vi "LucaStartAcquisition.vi"(5 "Camera Index":i32=1, 6 "Continuous":bool=TRUE, 7 "input cluster":T1={"left"=1, "right"=-1, "top"=1, "bottom"=-1}, 8 "error in (no error) 2":errorcluster, 9 "Bin Size":i32=1, 10 "EMCCD Gain":i32=200, 11 "Exposure Time":sgl=0.3 format="%.2f") -> (0 "error out":errorcluster={"status"=FALSE, "code"=0, "source"="LucaDetectIon.vi->LucaStartAcquisition.vi->SetShutter.vi"}, 3 "Image":u16[][](array[numeric]))   [LabVIEW 2009]
uses:
  <userlib>/atmcd32d.llb/AcquisitionMode_mode typedef.ctl
  <userlib>/atmcd32d.llb/ReadMode_mode typedef.ctl
  <userlib>/atmcd32d.llb/TriggerMode_mode typedef.ctl
  <userlib>/atmcd32d.llb/Shutter_mode typedef.ctl
  <userlib>/atmcd32d.llb/Shutter_type typedef.ctl
panel:
  out "Calculated Exposure Time":sgl=0.3 format="%.2f"
  out "Kinetic Cycle Time":sgl=0.3009 format="%.2f"
  out "Accumulate Time":sgl=0.3009 format="%.2f"
  out "Set Trigger Mode\nError Code":u32=20002
  out "Camera Serial":i32=1151
  out "Initialize Error Code":u32=20002
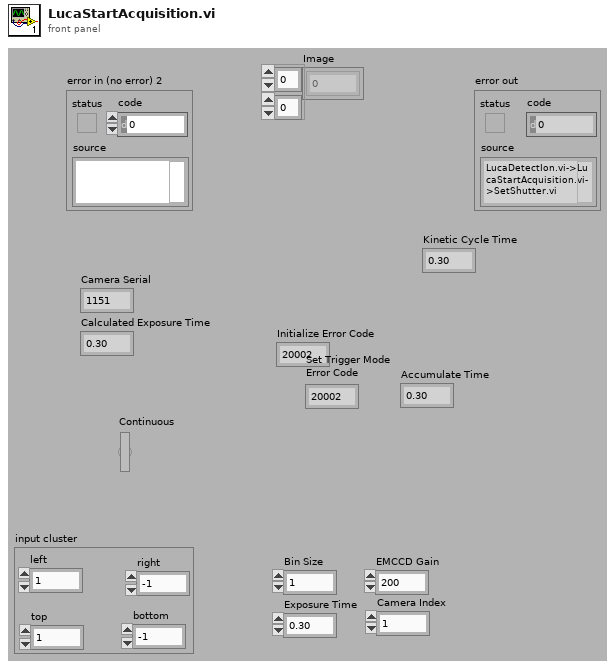
[diagram p1: front panel]
types:
  T1 = cluster{"left":i32, "right":i32, "top":i32, "bottom":i32}
  T2 = typedef "AcquisitionMode_mode typedef.ctl" = enum16{"Reserved (0)", "Single Scan", "Accumulate", "Kinetics", "Fast Kinetics", "Run Till Abort", "Reserved (6)", "Reserved (7)", "Reserved (8)", "Time Delayed Integration"}
  T3 = typedef "ReadMode_mode typedef.ctl" = enum16{"Full Vertical Binning", "Multi-Track", "Random-Track", "Single-Track", "Image"}
  T4 = typedef "TriggerMode_mode typedef.ctl" = enum16{"Internal", "External", "N/A (2)", "N/A (3)", "N/A (4)", "N/A (5)", "External Start"}
  T5 = typedef "Shutter_mode typedef.ctl" = enum16{"Auto", "Open", "Close"}
  T6 = typedef "Shutter_type typedef.ctl" = enum16{"TTL Low", "TTL High"}
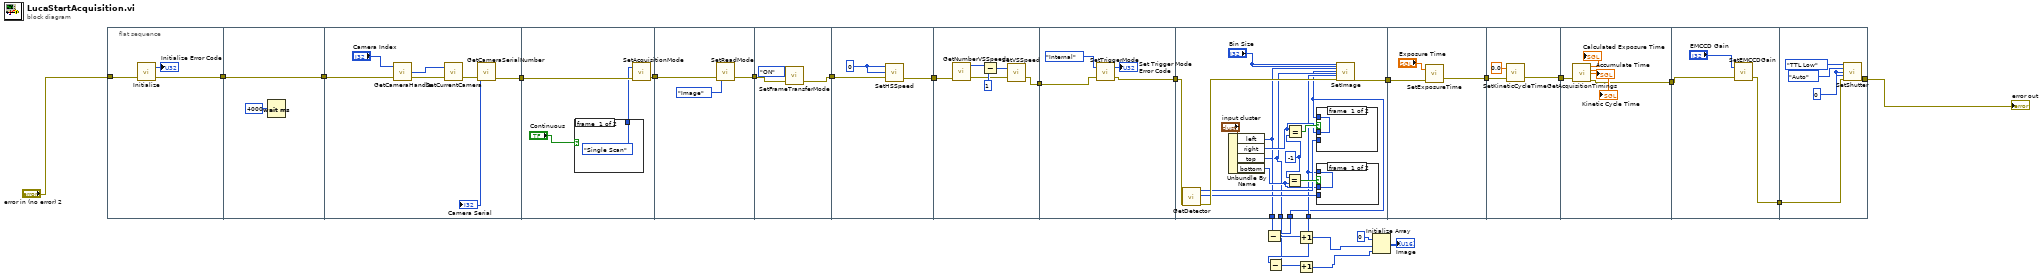
[diagram p0: block diagram]
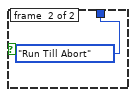
[diagram p2: hidden frame]
diagram:
  n1 = flat-sequence {
    tunnel: [w28] -> w26
    tunnel: "error in (no error) 2" -> [w27]
    tunnel: [w30] -> w25
    tunnel: w26 -> [w30]
    tunnel: [w33] -> w24
    tunnel: w25 -> [w32]
    tunnel: w24 -> [w42]
    tunnel: [w41] -> w23
    tunnel: w23 -> [w46]
    tunnel: [w45] -> w6
    tunnel: w6 -> [w50]
    tunnel: [w49] -> w5
    tunnel: w5 -> [w52]
    tunnel: [w51] -> w22
    tunnel: w22 -> [w56]
    tunnel: [w54] -> w21
    tunnel: w21 -> [w60]
    tunnel: [w61] -> w20
    tunnel: w20 -> [w78]
    tunnel: [w76] -> w19
    tunnel: [w67] -> w9
    tunnel: [w66] -> w7
    tunnel: [w65] -> w8
    tunnel: [w64] -> w10
    tunnel: w19 -> [w85]
    tunnel: [w84] -> w18
    tunnel: w18 -> [w89]
    tunnel: [w88] -> w17
    tunnel: w17 -> [w93]
    tunnel: [w90] -> w16
    tunnel: [w96] -> w15
    tunnel: w16 -> [w95]
    tunnel: w15 -> [w100]
    tunnel: [w98] -> w14
    frame #0 {
      n2 = call <userlib>:"Initialize.vi"("error in (no error)"=w27) -> ("error out"=w28:errorcluster, "DLL error code"=→"Initialize Error Code":u32)  [unwired: 1 in]
    }
    frame #1 {
      n3 = Wait (ms)(milliseconds to wait=u32 4000) -> ()  [unwired: 1 out]
    }
    frame #2 {
      n4 = call <userlib>:"GetCameraHandle.vi"("error in (no error)"=w32, "cameraIndex"="Camera Index") -> ("error out"=w38:errorcluster, "cameraHandle"=w37:i32)  [unwired: 1 in, 1 out]
      n5 = call <userlib>:"SetCurrentCamera.vi"("error in (no error)"=w38, "cameraHandle"=w37) -> ("error out"=w35:errorcluster)  [unwired: 1 out]
      n6 = call <userlib>:"GetCameraSerialNumber.vi"("error in (no error)"=w35) -> ("error out"=w33:errorcluster, "number"=→"Camera Serial":i32)  [unwired: 2 in, 1 out]
    }
    frame #3 {
      n7 = case shown="False" "Continuous" {
        tunnel: [AcquisitionMode_mode_typedef."Single Scan" ("mode") AcquisitionMode_mode_typedef."Run Till Abort" ("mode")] -> w39
        frame #0 {
        }
        frame #1 {
        }
      }
      n8 = call <userlib>:"SetAcquisitionMode.vi"("error in (no error)"=w42, "mode"=w39) -> ("error out"=w41:errorcluster)  [unwired: 1 out]
    }
    frame #4 {
      n9 = call <userlib>:"SetReadMode.vi"("error in (no error)"=w46, "mode"=ReadMode_mode_typedef."Image") -> ("error out"=w45:errorcluster)  [unwired: 1 out]
    }
    frame #5 {
      n10 = call <userlib>:"SetFrameTransferMode.vi"("error in (no error)"=w50, "mode"=enum16{"OFF", "ON"}."ON") -> ("error out"=w49:errorcluster)  [unwired: 1 out]
    }
    frame #6 {
      w53 = 0
      n11 = call <userlib>:"SetHSSpeed.vi"("error in (no error)"=w52, "index"=w53, "type"=w53) -> ("error out"=w51:errorcluster)  [unwired: 1 in, 1 out]
    }
    frame #7 {
      n12 = call <userlib>:"GetNumberVSSpeeds.vi"("error in (no error)"=w56) -> ("error out"=w55:errorcluster, "number"=w59:i32)  [unwired: 2 in, 1 out]
      n13 = Subtract(x=w59, y=1) -> (x-y=w57:i32)
      n14 = call <userlib>:"SetVSSpeed.vi"("error in (no error)"=w55, "index"=w57) -> ("error out"=w54:errorcluster)  [unwired: 1 out]
    }
    frame #8 {
      n15 = call <userlib>:"SetTriggerMode.vi"("error in (no error)"=w60, "mode"=TriggerMode_mode_typedef."Internal") -> ("error out"=w61:errorcluster, "DLL error code"=→"Set Trigger Mode\nError Code":u32)
    }
    frame #9 {
      w72 = -1
      n16 = call <userlib>:"GetDetector.vi"("error in (no error)"=w78) -> ("error out"=w77:errorcluster, "ypixels"=w71:i32, "xpixels"=w70:i32)  [unwired: 3 in, 1 out]
      n17 = Unbundle By Name("input cluster") -> ("left"=w67:i32, "right"=w69:i32, "top"=w66:i32, "bottom"=w68:i32)
      n18 = Equal?(x=w72, y=w68) -> (x = y?=w73:bool)
      n19 = Equal?(x=w69, y=w72) -> (x = y?=w74:bool)
      n20 = case shown="True" w74 {
        tunnel: [w82 w83] -> w64
        tunnel: w70 -> [_ w83]
        tunnel: w69 -> [w82 _]
        frame #0 {
        }
        frame #1 {
        }
      }
      n21 = case shown="True" w73 {
        tunnel: [w80 w81] -> w65
        tunnel: w71 -> [_ w81]
        tunnel: w68 -> [w80 _]
        frame #0 {
        }
        frame #1 {
        }
      }
      n22 = call <userlib>:"SetImage.vi"("hbin"="Bin Size", "vbin"="Bin Size", "hstart"=w67, "hend"=w64, "vstart"=w66, "vend"=w65, "error in (no error)"=w77) -> ("error out"=w76:errorcluster)  [unwired: 19 in, 1 out]
    }
    frame #10 {
      n23 = call <userlib>:"SetExposureTime.vi"("error in (no error)"=w85, "time"="Exposure Time") -> ("error out"=w84:errorcluster)  [unwired: 1 out]
    }
    frame #11 {
      n24 = call <userlib>:"SetKineticCycleTime.vi"("error in (no error)"=w89, "time"=sgl 0.0) -> ("error out"=w88:errorcluster)  [unwired: 1 out]
    }
    frame #12 {
      n25 = call <userlib>:"GetAcquisitionTimings.vi"("error in (no error)"=w93) -> ("exposure"=→"Calculated Exposure Time":sgl, "accumulate"=→"Accumulate Time":sgl, "kinetic"=→"Kinetic Cycle Time":sgl, "error out"=w90:errorcluster)  [unwired: 10 in, 1 out]
    }
    frame #13 {
      n26 = call <userlib>:"SetEMCCDGain.vi"("error in (no error)"=w95, "gain"="EMCCD Gain") -> ("error out"=w96:errorcluster)  [unwired: 1 out]
    }
    frame #14 {
      w99 = 0 ("closingtime")
      n27 = call <userlib>:"SetShutter.vi"("type"=Shutter_type_typedef."TTL Low", "mode"=Shutter_mode_typedef."Auto", "closingtime"=w99, "openingtime"=w99, "error in (no error)"=w100) -> ("error out"=w98:errorcluster)  [unwired: 9 in, 1 out]
    }
  }
  n28 = Subtract(x=w10, y=w9) -> (x-y=w11:i32)
  n29 = Subtract(x=w8, y=w7) -> (x-y=w12:i32)
  n30 = Increment(x=w11) -> (x+1=w3:i32)
  n31 = Increment(x=w12) -> (x+1=w2:i32)
  n32 = Initialize Array(u16 0, w3, w2) -> (→"Image":u16[][])
  "error out" <- w14
